vi "UHR-Fleezers Control (host) - Lorentz v5.vi"() -> ()   [LabVIEW 2014] (continued)
            "Current Position" <- w771
            n450 = local write "Stage Control Serial Error"(w774) -> ()
            n451 = Unbundle(w771) -> (w778:dbl, w780:dbl, w776:dbl)
            n452 = Add(x=w780, y="Y change (mm)") -> (x+y=w777:dbl)
            n453 = Bundle(w778, w777, w776) -> (w775:cluster{dbl, dbl, dbl})  [unwired: 1 in]
          }
          frame #1 {
            # "move to new position and start saving"
            n454 = local write "Stage Moving"(TRUE ("Stage Moving")) -> ()
            n455 = local write "Start Saving"(TRUE ("Start Saving")) -> ()
            n456 = call "Set Stage Position.vi"("Position"=w788, "error in"=w787, "VISA resource name in"=w786) -> ("error out"=w784:errorcluster, "VISA resource name out"=w785:refnum<visa-resource-name>)  [unwired: 1 out]
          }
          frame #2 {
            # "go back to start"
            n457 = call "Set Stage Position.vi"("Position"=w790, "error in"=w791, "VISA resource name in"=w792) -> ()  [unwired: 3 out]
          }
          frame #3 {
            # "stop saving"
            n458 = local write "Stop Saving"(TRUE ("Stop Saving")) -> ()
            n459 = local write "Stage Moving"(FALSE ("Stage Moving")) -> ()
          }
        }
      }
      event "Move to Position 1", "Move to Position 2", "Move to Position 3", "Move to Position 4", "Move to Position 5", "Lower Ch. Cap.", "Move to Position 6": Value Change {
        n460 = event-data() -> ()  [unwired: 1 in, 5 out]
        n461 = Or(x="Move to Position 5", y="Lower Ch. Cap.") -> (x .or. y?=w799:bool)
        n462 = Build Array("Move to Position 1", "Move to Position 2", "Move to Position 3", "Move to Position 4", w799, "Move to Position 6") -> (w802:bool[])
        n463 = Boolean Array To Number(Boolean array=w802) -> (number=w801:u32)
        n464 = Logarithm Base 2(1:w801) -> (0:w800:dbl)
        n465 = flat-sequence {
          tunnel: w800 -> [w811]
          tunnel: w797 -> [w809]
          tunnel: w796 -> [w808]
          frame #0 {
            n466 = local read "Saved Stage Positions"() -> (w819:dbl[][])
            n467 = Array Subset(array=w819, index (row)=w811, length (row)=1 ("length"), index (col)=1 ("index"), length (col)=3 ("length")) -> (w816:dbl[][])
            n468 = Reshape Array(w816, 3 ("dimension size")) -> (w814:dbl[])
            n469 = Array To Cluster(array=w814) -> (cluster=w813:cluster{"[0]":dbl, "[1]":dbl, "[2]":dbl})
            n470 = call "Set Stage Position.vi"("Position"=w813, "error in"=w808, "VISA resource name in"=w809) -> ("error out"=w812:errorcluster)  [unwired: 2 out]
            n471 = local write "Stage Moving"(TRUE ("Stage Moving")) -> ()
            n472 = local write "Stage Control Serial Error"(w812) -> ()
          }
          frame #1 {
            n473 = local write "Stage Moving"(FALSE ("Stage Moving")) -> ()
            n474 = call <vilib>:"Beep.vi"() -> ()  [unwired: 3 in, 9 out]
          }
        }
      }
      event "Got Bead 1": Value Change {
        n475 = event-data() -> ()  [unwired: 1 in, 5 out]
        n476 = flat-sequence {
          tunnel: w822 -> [w824]
          tunnel: w822 -> [w828]
          frame #0 {
            n477 = for {
              N: w824 -> [_]
              n478 = property on="Pressure Up" class="Bool (strict)"("Val(Sgnl)"=TRUE) -> ()  [unwired: 2 in, 2 out]
            }
          }
          frame #1 {
          }
          frame #2 {
            n479 = Wait (ms)(milliseconds to wait=u32 1000) -> ()  [unwired: 1 out]
          }
          frame #3 {
          }
          frame #4 {
            n480 = Multiply(x=w828, y=2) -> (x*y=w827:i32)
            n481 = for {
              N: w827 -> [_]
              n482 = property on="Vent pressure" class="Bool (strict)"("Val(Sgnl)"=TRUE) -> ()  [unwired: 2 in, 2 out]
            }
          }
          frame #5 {
            n483 = for {
              N: "Number of Pulses for bead 2" -> [_]
              n484 = property on="Pressure Up" class="Bool (strict)"("Val(Sgnl)"=TRUE) -> ()  [unwired: 2 in, 2 out]
            }
          }
        }
        n485 = local read "Number of pulses For laminar flow"() -> (w822:i32)
      }
      event "Force FB Data\nScript": Value Change {
        n486 = event-data() -> ()  [unwired: 1 in, 5 out]
        n487 = flat-sequence {
          tunnel: w838 -> [w842]
          tunnel: w839 -> [w843]
          tunnel: [w843] -> w834
          tunnel: [w842] -> w833
          tunnel: w834 -> [w846]
          tunnel: w833 -> [w845]
          tunnel: ["Trap Trig Fl."] -> w835
          tunnel: [w871] -> w836
          tunnel: w835 -> [w871]
          tunnel: [w875] -> w837
          tunnel: w836 -> [w875]
          tunnel: w837 -> [w877]
          frame #0 {
            n488 = property on="Trap Delta (MHz)" class="DigNum (strict)"("Val(Sgnl)"="Trap Delta Before Moving") -> ()  [unwired: 2 in, 2 out]
          }
          frame #1 {
            n489 = local read "Saved Stage Positions"() -> (w848:dbl[][])
            n490 = property on="Trap Pos. FB Offset Factor" class="DigNum (strict)"("Val(Sgnl)"=i64 0 ("Value (Signaling)")) -> ()  [unwired: 2 in, 2 out]
            n491 = local write "FB Trap Pos Offset"(0.0 ("FB Trap Pos Offset")) -> ()
            n492 = local write "Stage Moving"(TRUE ("Stage Moving")) -> ()
            n493 = call "move to saved stage position.vi"("error in"=w845, "Stage VISA resource name in"=w846, "Position"="Stage Position To Establish FB", "Saved Stage Positions"=w848) -> ("error out"=w844:errorcluster)  [unwired: 1 out]
            n494 = local write "Stage Control Serial Error"(w844) -> ()
          }
          frame #2 {
            n495 = call <vilib>:"Beep.vi"() -> ()  [unwired: 3 in, 9 out]
            n496 = Multiply(x="Wait (s)", y=u32 1000 ("milliseconds to wait")) -> (x*y=w855:u32)
            n497 = property on="Trap Delta (MHz)" class="DigNum (strict)"("Val(Sgnl)"="Starting \nTrap Delta (MHz)") -> ()  [unwired: 2 in, 2 out]
            n498 = local write "Stage Moving"(FALSE ("Stage Moving")) -> ()
            n499 = Wait (ms)(milliseconds to wait=w855) -> ()  [unwired: 1 out]
            n500 = property on="Tab Control 2" class="TabCtl (strict)"("Val(Sgnl)"=T11."Feedback on Trap Position" ("Value (Signaling)")) -> ()  [unwired: 2 in, 2 out]
            n501 = property on="Tab Control" class="TabCtl (strict)"("Val(Sgnl)"=T40."Trap Control (RF)" ("Value (Signaling)")) -> ()  [unwired: 2 in, 2 out]
          }
          frame #3 {
            n502 = property on="Set Reading to\nSetpoint" class="Bool (strict)"("Val(Sgnl)"=TRUE ("Value (Signaling)")) -> ()  [unwired: 2 in, 2 out]
            n503 = Wait (ms)(milliseconds to wait=u32 500) -> ()  [unwired: 1 out]
          }
          frame #4 {
            n504 = property on="Trap Pos. FB ON" class="Bool (strict)"("Val(Sgnl)"=TRUE ("Value (Signaling)")) -> ()  [unwired: 2 in, 2 out]
            n505 = Wait (ms)(milliseconds to wait=u32 250) -> ()  [unwired: 1 out]
          }
          frame #5 {
            n506 = case shown="False" "Trap Trig Fl." {
              frame False {
                n507 = case shown="True" "Green ON after FB ON?" {
                  selector: "Green ON after FB ON?" -> [_ w870]
                  frame False {
                  }
                  frame True {
                    n508 = property on="Green Laser ON" class="Bool (strict)"("Val(Sgnl)"=w870) -> ()  [unwired: 2 in, 2 out]
                  }
                }
              }
              frame True {
              }
            }
            n509 = case shown="True" "Remove Action Offset" {
              tunnel: TRUE ("Value (Signaling)") -> [w867 w868]
              frame False {
                n510 = property on="Remove Unwinding Offset" class="Bool (strict)"("Val(Sgnl)"=w867) -> ()  [unwired: 2 in, 2 out]
              }
              frame True {
                n511 = property on="Remove Action Offset" class="Bool (strict)"("Val(Sgnl)"=w868) -> ()  [unwired: 2 in, 2 out]
              }
            }
            n512 = Wait (ms)(milliseconds to wait=u32 250) -> ()  [unwired: 1 out]
          }
          frame #6 {
            n513 = property on="Start Saving" class="Bool (strict)"("Val(Sgnl)"=TRUE ("Value (Signaling)")) -> ()  [unwired: 2 in, 2 out]
            n514 = Wait (ms)(milliseconds to wait=u32 5000) -> ()  [unwired: 1 out]
          }
          frame #7 {
            w874 = TRUE ("Value (Signaling)")
            n515 = property on="Rem fb disp offset" class="Bool (strict)"("Val(Sgnl)"=w874) -> ()  [unwired: 2 in, 2 out]
            n516 = property on="Remove Offset" class="Bool (strict)"("Val(Sgnl)"=w874) -> ()  [unwired: 2 in, 2 out]
            n517 = Wait (ms)(milliseconds to wait=u32 100) -> ()  [unwired: 1 out]
          }
          frame #8 {
            n518 = case shown="True" w877 {
              frame False {
              }
              frame True {
                n519 = local write "Trap Trig. Fl."(TRUE ("Value (Signaling)")) -> ()
              }
            }
          }
          frame #9 {
            n520 = case shown="True" "Start dipping after?" {
              frame False {
              }
              frame True {
                n521 = flat-sequence {
                  frame #0 {
                    n522 = Multiply(x="Delay before dipping (s)", y=1000.0) -> (x*y=w881:dbl)
                    n523 = Wait (ms)(milliseconds to wait=w881) -> ()  [unwired: 1 out]
                  }
                  frame #1 {
                    n524 = property on="Dip for Protein" class="Bool (strict)"("Val(Sgnl)"=TRUE ("Value (Signaling)")) -> ()  [unwired: 2 in, 2 out]
                    n525 = local write "Scripts"(T2."Dipping" ("Scripts")) -> ()
                  }
                }
              }
            }
          }
        }
      }
      event "Fixed Traps Data\nScript": Value Change {
        n526 = event-data() -> ()  [unwired: 1 in, 5 out]
        n527 = flat-sequence {
          frame #0 {
            n528 = case shown="True" "Green ON" {
              frame False {
              }
              frame True {
                n529 = property on="Green Laser ON" class="Bool (strict)"("Val(Sgnl)"=TRUE) -> ()  [unwired: 2 in, 2 out]
              }
            }
            n530 = local write "Offset (nm)"(0.0 ("Offset (nm)")) -> ()
            n531 = property on="Sample Channel\nFlow" class="Bool (strict)"("Val(Sgnl)"=FALSE ("Value (Signaling)")) -> ()  [unwired: 2 in, 2 out]
            n532 = property on="Trap Delta (MHz)" class="DigNum (strict)"("Val(Sgnl)"="Fixed Traps Trap Delta (MHz)") -> ()  [unwired: 2 in, 2 out]
          }
          frame #1 {
            n533 = Wait (ms)(milliseconds to wait=u32 1000) -> ()  [unwired: 1 out]
          }
          frame #2 {
            n534 = local write "Start Saving"(TRUE ("Start Saving")) -> ()
          }
          frame #3 {
            n535 = local read "Bead Sep. Int. Time (s)"() -> (w892:dbl)
            n536 = Multiply(x=w892, y=1000.0) -> (x*y=w894:dbl)
            n537 = Wait (ms)(milliseconds to wait=w894) -> ()  [unwired: 1 out]
          }
          frame #4 {
            n538 = property on="Remove Offset" class="Bool (strict)"("Val(Sgnl)"=TRUE ("Value (Signaling)")) -> ()  [unwired: 2 in, 2 out]
          }
          frame #5 {
            n539 = property on="Dip for Protein" class="Bool (strict)"("Val(Sgnl)"="Start dipping after?") -> ()  [unwired: 2 in, 2 out]
          }
        }
      }
      event "Got Bead 2": Value Change {
        # "Got A Dig bead and Got DNA bead events changes by Ronen to Got bead 1 and Got bead 2, and modified to enable operation of the thorlabs motors."
        n540 = event-data() -> ()  [unwired: 1 in, 5 out]
        n541 = flat-sequence {
          tunnel: w897 -> [w900]
          frame #0 {
            n542 = case shown="True" "Lumicks Flow During Calibration" {
              tunnel: w900 -> [_ w901]
              frame False {
              }
              frame True {
                n543 = for {
                  N: w901 -> [_]
                  n544 = property on="Pressure Up" class="Bool (strict)"("Val(Sgnl)"=TRUE) -> ()  [unwired: 2 in, 2 out]
                }
              }
            }
          }
          frame #1 {
          }
          frame #2 {
            n545 = Wait (ms)(milliseconds to wait=u32 1000) -> ()  [unwired: 1 out]
          }
          frame #3 {
          }
          frame #4 {
            n546 = case shown="True" "Calibrate after bead 2?" {
              frame False {
              }
              frame True {
                n547 = property on="Cal/Data Acq. Spot" class="Bool (strict)"("Val(Sgnl)"=TRUE) -> ()  [unwired: 2 in, 2 out]
              }
            }
          }
        }
        n548 = local read "Number of pulses For laminar flow"() -> (w897:i32)
      }
      event "Get New Beads": Value Change {
        # "Flow Control determines how many pressure increases are given when moving."
        n549 = event-data() -> ()  [unwired: 1 in, 6 out]
        n550 = flat-sequence {
          tunnel: w906 -> [w908]
          tunnel: w906 -> [w912]
          frame #0 {
            n551 = for {
              N: w908 -> [_]
              n552 = property on="Pressure Up" class="Bool (strict)"("Val(Sgnl)"=TRUE) -> ()  [unwired: 2 in, 2 out]
            }
          }
          frame #1 {
          }
          frame #2 {
            n553 = Wait (ms)(milliseconds to wait=u32 1000) -> ()  [unwired: 1 out]
          }
          frame #3 {
          }
          frame #4 {
            n554 = Multiply(x=2, y=w912) -> (x*y=w911:i32)
            n555 = for {
              N: w911 -> [_]
              n556 = property on="Vent pressure" class="Bool (strict)"("Val(Sgnl)"=TRUE) -> ()  [unwired: 2 in, 2 out]
            }
          }
          frame #5 {
            n557 = for {
              N: "Number of pulses for Bead 1" -> [_]
              n558 = property on="Pressure Up" class="Bool (strict)"("Val(Sgnl)"=TRUE) -> ()  [unwired: 2 in, 2 out]
            }
          }
        }
        n559 = local read "Number of pulses For laminar flow"() -> (w906:i32)
      }
      event "Take Stepping Data": Value Change {
        n560 = event-data() -> ()  [unwired: 1 in, 5 out]
        n561 = local read "Save ave N"() -> (w925:dbl)
        n562 = flat-sequence {
          tunnel: w925 -> [w927]
          tunnel: [w927] -> w920
          tunnel: [w929] -> w921
          tunnel: w920 -> [w929]
          tunnel: [w931] -> w922
          tunnel: w921 -> [w931]
          tunnel: [w934] -> w923
          tunnel: w922 -> [w934]
          tunnel: [w936] -> w924
          tunnel: w923 -> [w936]
          tunnel: [w938] -> w918
          tunnel: w924 -> [w938]
          tunnel: w918 -> [w941]
          tunnel: [w941] -> w917
          tunnel: w917 -> [w942]
          tunnel: [w942] -> w919
          tunnel: w919 -> [w948]
          frame #0 {
            n563 = property on="Save ave N" class="DigNum (strict)"("Val(Sgnl)"="Save ave factor") -> ()  [unwired: 2 in, 2 out]
          }
          frame #1 {
            n564 = Wait (ms)(milliseconds to wait=u32 100) -> ()  [unwired: 1 out]
          }
          frame #2 {
            n565 = local read "Offset 2 Start (MHz)"() -> (w933:dbl)
            n566 = property on="Saved AOD Raster Scan Parameter Sets" class="Arr (strict)"("Index Values"=u32[] [2]) -> ()  [unwired: 2 in, 2 out]
            n567 = property on="Trap Delta (MHz)" class="DigNum (strict)"("Val(Sgnl)"=w933) -> ()  [unwired: 2 in, 2 out]
          }
          frame #3 {
            n568 = property on="Load parameters" class="Bool (strict)"("Val(Sgnl)"=TRUE ("Value (Signaling)")) -> ()  [unwired: 2 in, 2 out]
          }
          frame #4 {
            n569 = Wait (ms)(milliseconds to wait=u32 100) -> ()  [unwired: 1 out]
          }
          frame #5 {
            n570 = property on="Trap Raster Scan" class="Bool (strict)"("Val(Sgnl)"=TRUE ("Value (Signaling)")) -> ()  [unwired: 2 in, 2 out]
          }
          frame #6 {
            n571 = Wait (ms)(milliseconds to wait=u32 1000) -> ()  [unwired: 1 out]
          }
          frame #7 {
            n572 = while {
              stop <- w945 stop-if-true
              n573 = local read "Raster Scanning..."() -> (w947:bool)
              n574 = local read "Saving..."() -> (w946:bool)
              n575 = Not(x=w946) -> (.not. x?=w943:bool)
              n576 = Not(x=w947) -> (.not. x?=w944:bool)
              n577 = And(x=w944, y=w943) -> (x .and. y?=w945:bool)
            }
          }
          frame #8 {
            n578 = property on="Save ave N" class="DigNum (strict)"("Val(Sgnl)"=w948) -> ()  [unwired: 2 in, 2 out]
          }
        }
      }
      event "Step Size (nm)": Value Change {
        n579 = event-data() -> ()  [unwired: 1 in, 5 out]
        n580 = flat-sequence {
          frame #0 {
            n581 = property on="Saved AOD Raster Scan Parameter Sets" class="Arr (strict)"("Index Values"=u32[] [1]) -> ()  [unwired: 2 in, 2 out]
          }
          frame #1 {
            n582 = Multiply(x="N Steps", y="Step Size (nm)") -> (x*y=w950:dbl)
            n583 = property on="Scan Speed AOD (nm/s) 2" class="DigNum (strict)"("Value"="Step Size (nm)") -> ()  [unwired: 2 in, 2 out]
            n584 = property on="Step Size AOD (nm) 2" class="DigNum (strict)"("Value"="Step Size (nm)") -> ()  [unwired: 2 in, 2 out]
            n585 = property on="Scan Range AOD (nm) 2" class="DigNum (strict)"("Value"=w950) -> ()  [unwired: 2 in, 2 out]
          }
        }
      }
      event "Take Detection Laser\nImage": Value Change {
        n586 = event-data() -> ()  [unwired: 1 in, 5 out]
        n587 = flat-sequence {
          tunnel: [w978] -> w968
          tunnel: [w977] -> w961
          tunnel: [w976] -> w953
          tunnel: [w981] -> w969
          tunnel: w968 -> [w981]
          tunnel: [w980] -> w962
          tunnel: w961 -> [w980]
          tunnel: [w979] -> w954
          tunnel: w953 -> [w979]
          tunnel: [w985] -> w970
          tunnel: w969 -> [w985]
          tunnel: [w984] -> w963
          tunnel: w962 -> [w984]
          tunnel: [w983] -> w955
          tunnel: w954 -> [w983]
          tunnel: [w991] -> w971
          tunnel: w970 -> [w991]
          tunnel: [w990] -> w964
          tunnel: w963 -> [w990]
          tunnel: [w989] -> w956
          tunnel: w955 -> [w989]
          tunnel: [w995] -> w972
          tunnel: w971 -> [w995]
          tunnel: [w994] -> w965
          tunnel: w964 -> [w994]
          tunnel: [w993] -> w957
          tunnel: w956 -> [w993]
          tunnel: [w999] -> w973
          tunnel: w972 -> [w999]
          tunnel: [w998] -> w966
          tunnel: w965 -> [w998]
          tunnel: [w997] -> w958
          tunnel: w957 -> [w997]
          tunnel: [w1003] -> w974
          tunnel: w973 -> [w1003]
          tunnel: [w1002] -> w967
          tunnel: w966 -> [w1002]
          tunnel: [w1001] -> w959
          tunnel: w958 -> [w1001]
          tunnel: w974 -> [w1009]
          tunnel: w967 -> [w1008]
          tunnel: [w1006] -> w960
          tunnel: w959 -> [w1006]
          tunnel: w960 -> [w1010]
          frame #0 {
            n588 = local read "Laser interlacing mode"() -> (w977:enum32{"Laser ON", "Laser OFF", "Interlace"})
            n589 = local read "Green FB On/Off"() -> (w976:bool)
            n590 = local read "Green Laser ON"() -> (w978:bool)
          }
          frame #1 {
            n591 = property on="Green FB On/Off" class="Bool (strict)"("Val(Sgnl)"=FALSE ("Value (Signaling)")) -> ()  [unwired: 2 in, 2 out]
          }
          frame #2 {
            n592 = property on="Green Laser ON" class="Bool (strict)"("Val(Sgnl)"=TRUE ("Value (Signaling)")) -> ()  [unwired: 2 in, 2 out]
            n593 = property on="Flip Green Filter" class="Bool (strict)"("Val(Sgnl)"=TRUE ("Value (Signaling)")) -> ()  [unwired: 2 in, 2 out]
            n594 = property on="Laser interlacing mode" class="RadioBtnsControl (strict)"("Val(Sgnl)"=enum32{"Laser ON", "Laser OFF", "Interlace"}."Laser ON" ("Value (Signaling)")) -> ()  [unwired: 2 in, 2 out]
          }
          frame #3 {
            n595 = Wait (ms)(milliseconds to wait=u32 500) -> ()  [unwired: 1 out]
          }
          frame #4 {
            n596 = property on="Confocal Image" class="Bool (strict)"("Val(Sgnl)"=TRUE ("Value (Signaling)")) -> ()  [unwired: 2 in, 2 out]
          }
          frame #5 {
            n597 = Wait (ms)(milliseconds to wait=u32 2000) -> ()  [unwired: 1 out]
          }
          frame #6 {
            n598 = while {
              stop <- w1004 stop-if-true
              n599 = local read "Saving..."() -> (w1005:bool)
              n600 = Not(x=w1005) -> (.not. x?=w1004:bool)
            }
          }
          frame #7 {
            n601 = property on="Flip Green Filter" class="Bool (strict)"("Val(Sgnl)"=TRUE ("Value (Signaling)")) -> ()  [unwired: 2 in, 2 out]
            n602 = property on="Green Laser ON" class="Bool (strict)"("Val(Sgnl)"=w1009) -> ()  [unwired: 2 in, 2 out]
            n603 = property on="Laser interlacing mode" class="RadioBtnsControl (strict)"("Val(Sgnl)"=w1008) -> ()  [unwired: 2 in, 2 out]
          }
          frame #8 {
            n604 = property on="Green FB On/Off" class="Bool (strict)"("Val(Sgnl)"=w1010) -> ()  [unwired: 2 in, 2 out]
          }
        }
      }
      event "Move in a Circle": Value Change {
        w1012 = dbl[] []
        # "converting distance (d) to angle (a)\na=arcsin(d/2r)"
        # "radius"
        # "radius"
        # "T1 Y"
        # "T1 X"
        n605 = event-data() -> ()  [unwired: 1 in, 5 out]
        n606 = local read "BD 1 Frequency 1 (MHz)"() -> (w1020:dbl)
        n607 = local read "BD 2 Frequency 1 (MHz)"() -> (w1019:dbl)
        n608 = local read "BD 1 Frequency 2 (MHz)"() -> (w1018:dbl)
        n609 = local read "BD 2 Frequency 2 (MHz)"() -> (w1017:dbl)
        n610 = Subtract(x=w1019, y="Center Y Frequency (MHz)") -> (x-y=w1024:dbl)
        n611 = Absolute Value(x=w1024) -> (abs(x)=w1015:dbl)
        n612 = flat-sequence {
          tunnel: w1015 -> [w1027]
          tunnel: [w1027] -> w1014
          frame #0 {
            n613 = local write "Radius (MHz)"(w1027) -> ()
          }
        }
        n614 = node-c288("Time step (ms)") -> (w1026:T36)  [unwired: 3 in]
        n615 = timed-loop {
          timing: w1026 -> [_]
          timing-out: [_] -> w1025
          tunnel: w1020 -> [w1118]
          tunnel: w1019 -> [_]
          tunnel: w1018 -> [w1122]
          tunnel: w1017 -> [_]
          tunnel: "Center Y Frequency (MHz)" -> [w1111]
          shift-right: [w1072] -> _
          shift-left: w1012 -> [w1079]
          shift-right: [w1070] -> _
          shift-left: w1012 -> [w1078]
          shift-right: [w1063] -> _
          shift-left: w1012 -> [w1076]
          shift-right: [w1061] -> _
          shift-left: w1012 -> [w1075]
          tunnel: "Move in a Circle" -> [_]
          tunnel: ["Back to start on finish?"] -> w1016
          tunnel: w1014 -> [_]
          tunnel: w1013 -> [w1093]
          tunnel: w1012 -> [w1074]
          shift-right: [w1045] -> _
          shift-left: 0.0 -> [w1043]
          i -> [w1052]
          stop <- w1116 stop-if-true
          w1060 = 0 ("index")
          w1081 = 1 ("dimension size")
          # "Keep phase within\n2pi so errors don't \nbuild"
          # "Accumulated\nphase"
          # "Current phase"
          # "Trap 2"
          # "Trap 1"
          # "ignore if N = 0"
          # "r"
          # "r"
          # "r"
          # "r"
          # "\"omega*t\""
          # "Trap 2"
          # "Trap separation (radians)"
          # "Trap 1"
          # "Offset (starts\n at bottom of\n the circle)"
          # "omega"
          n616 = node-c288() -> (w1129:i64)  [unwired: 1 in]
          n617 = Divide(x=w1129, y=1000) -> (x/y=w1048:dbl)
          n618 = Divide(x="2D Motion Trap Separation (MHz)", y="Radius (MHz)") -> (x/y=w1103:dbl)
          n619 = Negate(x=w1048) -> (-x=w1047:dbl)
          n620 = Divide(x="Trap 2 phase shift (deg)", y=360.0) -> (x/y=w1094:dbl)
          n621 = Inverse Sine(1:w1103) -> (0:w1039:dbl)
          n622 = Multiply(x=6.283185307179586, y=w1094) -> (x*y=w1040:dbl)
          n623 = Multiply(x=6.283185307179586, y="2D Motion Frequency (Hz)") -> (x*y=w1051:dbl)
          n624 = Select(t=w1048, s="Counterclockwise/Clockwise", f=w1047) -> (s? t:f=w1050:dbl)
          n625 = Multiply(x=w1051, y=w1050) -> (x*y=w1041:dbl)
          n626 = Select(t=w1039, s="Trap shift\nmethod", f=w1040) -> (s? t:f=w1038:dbl)
          n627 = Add(x=w1041, y=w1043) -> (x+y=w1044:dbl)
          n628 = Add(x=w1044, y=w1038) -> (x+y=w1100:dbl)
          n629 = Add(x=w1044, y=1.5707963267948966) -> (x+y=w1049:dbl)
          n630 = Add(x=w1100, y=1.5707963267948966) -> (x+y=w1113:dbl)
          n631 = Cosine(x=w1049) -> (cos(x)=w1127:dbl)
          n632 = Sine(x=w1049) -> (sin(x)=w1126:dbl)
          n633 = Multiply(x=w1127, y="Radius (MHz)") -> (x*y=w1120:dbl)
          n634 = Cosine(x=w1113) -> (cos(x)=w1125:dbl)
          n635 = Sine(x=w1113) -> (sin(x)=w1124:dbl)
          n636 = Multiply(x=w1126, y="Radius (MHz)") -> (x*y=w1119:dbl)
          n637 = Multiply(x=w1125, y="Radius (MHz)") -> (x*y=w1123:dbl)
          n638 = Multiply(x=w1124, y="Radius (MHz)") -> (x*y=w1121:dbl)
          n639 = Add(x=w1120, y=w1118) -> (x+y=w1069:dbl)
          n640 = Add(x=w1119, y=w1111) -> (x+y=w1067:dbl)
          n641 = Greater Or Equal?(x=w1052, y="N steps then stop") -> (x >= y?=w1110:bool)
          n642 = Add(x=w1123, y=w1122) -> (x+y=w1058:dbl)
          n643 = Add(x=w1121, y=w1111) -> (x+y=w1056:dbl)
          n644 = Not Equal To 0?(x="N steps then stop") -> (x != 0?=w1106:bool)
          n645 = And(x=w1110, y=w1106) -> (x .and. y?=w1107:bool)
          n646 = local read "Trap 1 sum mean"() -> (w1090:dbl)
          n647 = local read "Stop All"() -> (w1115:bool)
          n648 = local write "BD 1 Frequency 1 (MHz)"(w1069) -> ()
          n649 = local write "BD 2 Frequency 1 (MHz)"(w1067) -> ()
          n650 = local write "BD 1 Frequency 2 (MHz)"(w1058) -> ()
          n651 = local write "BD 2 Frequency 2 (MHz)"(w1056) -> ()
          n652 = Select(t=w1052, s="test", f=w1090) -> (s? t:f=→"Waveform Chart":dbl)
          n653 = Compound Arithmetic op=OR(w1115, "Stop Moving", w1107) -> (w1116:bool)
          n654 = local read "BD 1 Frequency 3 (MHz)"() -> (w1099:dbl)
          n655 = local read "BD 2 Frequency 3 (MHz)"() -> (w1098:dbl)
          n656 = Select(t=w1074, s="Reset graph", f=w1075) -> (s? t:f=w1055:dbl[])
          n657 = Select(t=w1074, s="Reset graph", f=w1076) -> (s? t:f=w1057:dbl[])
          n658 = Select(t=w1074, s="Reset graph", f=w1078) -> (s? t:f=w1066:dbl[])
          n659 = Select(t=w1074, s="Reset graph", f=w1079) -> (s? t:f=w1068:dbl[])
          n660 = Initialize Array(w1056, w1081) -> (w1082:dbl[])
          n661 = Initialize Array(w1067, w1081) -> (w1085:dbl[])
          n662 = Initialize Array(w1058, w1081) -> (w1083:dbl[])
          n663 = Initialize Array(w1069, w1081) -> (w1086:dbl[])
          n664 = local read "Y RF Frequency Limits (MHz)"() -> (w1096:T23)
          n665 = local read "X RF Frequency Limits (MHz)"() -> (w1097:T23)
          n666 = call "set RF board frequency - interlace.vi"("Board 2 Frequency Limits"=w1096, "Board 1 Frequency Limits"=w1097, "FPGA VI Reference In"=w1093, "Board 2 Frequency 3 (MHz)"=w1098, "Board 1 Frequency 3 (MHz)"=w1099, "Board 2 Frequency 2 (MHz)"=w1056, "Board 2 Frequency 1 (MHz)"=w1067, "Board 1 Frequency 2 (MHz)"=w1058, "Board 1 Frequency 1  (MHz)"=w1069) -> ()  [unwired: 1 in, 2 out]
          n667 = Bundle(w1083, w1082) -> (w1054:cluster{dbl[], dbl[]})  [unwired: 1 in]
          n668 = Bundle(w1086, w1085) -> (w1084:cluster{dbl[], dbl[]})  [unwired: 1 in]
          n669 = Build Array (concatenate)(w1069, w1068) -> (w1073:dbl[])
          n670 = Build Array (concatenate)(w1067, w1066) -> (w1071:dbl[])
          n671 = Build Array (concatenate)(w1058, w1057) -> (w1064:dbl[])
          n672 = Build Array (concatenate)(w1056, w1055) -> (w1062:dbl[])
          n673 = Bundle(w1073, w1071) -> (w1053:cluster{dbl[], dbl[]})  [unwired: 1 in]
          n674 = Bundle(w1064, w1062) -> (w1080:cluster{dbl[], dbl[]})  [unwired: 1 in]
          n675 = Build Array(w1084, w1054, w1053, w1080) -> (→"Trap trajectories":cluster{dbl[], dbl[]}[])
          n676 = case "To pause the process" shown="True" "Pause rotation" {
            frame False {
            }
            frame True {
              n677 = while {
                stop <- w1132 stop-if-true
                n678 = local read "Pause rotation"() -> (w1133:bool)
                n679 = Wait (ms)(milliseconds to wait=u32 10) -> ()  [unwired: 1 out]
                n680 = Not(x=w1133) -> (.not. x?=w1132:bool)
              }
            }
          }
          n681 = Decrement(x="N steps to plot") -> (x-1=w1059:i32)
          n682 = Array Subset(array=w1071, index=w1060, length=w1059) -> (w1070:dbl[])
          n683 = Array Subset(array=w1073, index=w1060, length=w1059) -> (w1072:dbl[])
          n684 = Array Subset(array=w1064, index=w1060, length=w1059) -> (w1063:dbl[])
          n685 = Array Subset(array=w1062, index=w1060, length=w1059) -> (w1061:dbl[])
          n686 = Quotient & Remainder(x=w1044, y=6.283185307179586) -> (x-y*floor(x/y)=w1045:dbl)  [unwired: 1 out]
          n687 = node-c288() -> ()  [unwired: 1 in, 1 out]
        }
        n688 = node-c288(w1025) -> ()  [unwired: 1 out]
        n689 = case shown="True" w1016 {
          tunnel: w1020 -> [_ w1031]
          tunnel: w1019 -> [_ w1030]
          tunnel: w1018 -> [_ w1029]
          tunnel: w1017 -> [_ w1028]
          frame False {
          }
          frame True {
            n690 = flat-sequence {
              tunnel: w1031 -> [w1035]
              tunnel: w1030 -> [w1034]
              tunnel: w1029 -> [w1033]
              tunnel: w1028 -> [w1032]
              frame #0 {
                n691 = local write "BD 1 Frequency 1 (MHz)"(w1035) -> ()
                n692 = local write "BD 2 Frequency 1 (MHz)"(w1034) -> ()
                n693 = local write "BD 1 Frequency 2 (MHz)"(w1033) -> ()
                n694 = local write "BD 2 Frequency 2 (MHz)"(w1032) -> ()
              }
              frame #1 {
                n695 = property on="Update all trap values" class="Bool (strict)"("Val(Sgnl)"=TRUE ("Value (Signaling)")) -> ()  [unwired: 2 in, 2 out]
              }
            }
          }
        }
      }
      event "Stop All": Value Change {
        # "Stopping blue laser before shutting off program"
        n696 = event-data() -> ()  [unwired: 1 in, 5 out]
        n697 = local read "Delay (ms)"() -> (w1143:i32)
        n698 = call "serial write macro.vi"("String"="l0", "Delay (ms)"=w1143, "VISA resource name"=w1146) -> ("read buffer"=w1141:string, "error out"=w1142:errorcluster, "VISA resource name out"=w1145:refnum<visa-resource-name>)
        n699 = local write "read blue buffer"(w1141) -> ()
        n700 = local write "Blue Error Out"(w1142) -> ()
        n701 = VISA Close(VISA resource name=w1145) -> ()  [unwired: 1 in, 1 out]
        n702 = local read "Stop All"() -> (w1147:bool)
      }
      event "Sensitivity", "Offset Current Sign", "Offset Current Value", "Offset Current", "Bias Voltage", "Bias Voltage (mV)", "Filter Type", "Lowpass 3dB Point", "Highpass 3dB Point", "Filter Reset", "Invert Signal", "Gain Mode", "Send Command": Value Change {
        w1154 = 250 ("Delay (ms)")
        n703 = event-data() -> ()  [unwired: 1 in, 5 out]
        n704 = event shown="[0] \"Sensitivity\": Value Change" {
          selector: _ -> [_ _ _ _ _ _ _ _ _ _ _ _ _]
          dyn-events: _ -> [_ _ _ _ _ _ _ _ _ _ _ _ _]
          timeout: _ -> [_ _ _ _ _ _ _ _ _ _ _ _ _]
          tunnel: [w1166 w1174 w1182 w1191 w1201 w1209 w1212 w1216 w1219 w1222 w1225 w1232 "Command"] -> w1153
          tunnel: [w1161 w1168 w1178 w1185 w1195 w1205 _ _ _ _ _ w1228 _] -> w1148
          event "Sensitivity": Value Change {
            n705 = event-data() -> ()  [unwired: 1 in, 5 out]
            n706 = property on="Sensitivity" class="CmbBox"() -> ("Value"=→"Gain":string)  [unwired: 2 in, 2 out]
            n707 = Concatenate Strings("SENS ", "Sensitivity") -> (w1166:string)
            n708 = local read "Gain"() -> (w1163:string)
            n709 = Concatenate Strings("gain set at ", w1163) -> (w1161:string)
          }
          event "Offset Current Sign": Value Change {
            n710 = event-data() -> ()  [unwired: 1 in, 4 out]
            n711 = Boolean To (0,1)(Boolean="Offset Current Sign") -> (0, 1=w1177:i16)
            n712 = Select(t="positive", s="Offset Current Sign", f="negative") -> (s? t:f=w1169:string)
            n713 = Number To Decimal String(number=w1177) -> (decimal integer string=w1176:string)  [unwired: 1 in]
            n714 = Concatenate Strings("IOSN " ("string"), w1176) -> (w1174:string)
            n715 = Concatenate Strings("offset current sign ", w1169) -> (w1168:string)
          }
          event "Offset Current Value": Value Change {
            n716 = event-data() -> ()  [unwired: 1 in, 5 out]
            n717 = property on="Offset Current Value" class="CmbBox"() -> ("Value"=→"Read offset current":string)  [unwired: 2 in, 2 out]
            n718 = local read "Read offset current"() -> (w1179:string)
            n719 = Concatenate Strings("IOLV ", "Offset Current Value") -> (w1182:string)
            n720 = Concatenate Strings("offset current value ", w1179) -> (w1178:string)
          }
          event "Offset Current": Value Change {
            n721 = event-data() -> ()  [unwired: 1 in, 5 out]
            n722 = Boolean To (0,1)(Boolean="Offset Current") -> (0, 1=w1194:i16)
            n723 = Select(t="on", s="Offset Current", f="off") -> (s? t:f=w1186:string)
            n724 = Number To Decimal String(number=w1194) -> (decimal integer string=w1193:string)  [unwired: 1 in]
            n725 = Concatenate Strings("IOON " ("string"), w1193) -> (w1191:string)
            n726 = Concatenate Strings("offset current ", w1186) -> (w1185:string)
          }
          event "Bias Voltage": Value Change {
            n727 = event-data() -> ()  [unwired: 1 in, 5 out]
            n728 = Boolean To (0,1)(Boolean="Bias Voltage") -> (0, 1=w1202:i16)
            n729 = Number To Decimal String(number=w1202) -> (decimal integer string=w1203:string)  [unwired: 1 in]
            n730 = Select(t="on", s="Bias Voltage", f="off") -> (s? t:f=w1196:string)
            n731 = Concatenate Strings("BSON " ("string"), w1203) -> (w1201:string)
            n732 = Concatenate Strings("bias voltage", w1196) -> (w1195:string)
          }
          event "Bias Voltage (mV)": Value Change {
            n733 = event-data() -> ()  [unwired: 1 in, 5 out]
            n734 = Number To Decimal String(number="Bias Voltage (mV)") -> (decimal integer string=w1211:string)  [unwired: 1 in]
            n735 = Number To Fractional String(number="Bias Voltage (mV)") -> (F-format string=w1206:string)  [unwired: 3 in]
            n736 = Concatenate Strings("BSLV " ("string"), w1211) -> (w1209:string)
            n737 = Concatenate Strings("bias voltage value ", w1206) -> (w1205:string)
          }
          event "Filter Type": Value Change {
            n738 = event-data() -> ()  [unwired: 1 in, 5 out]
            n739 = Concatenate Strings("FLTT " ("string"), "Filter Type") -> (w1212:string)
          }
          event "Lowpass 3dB Point": Value Change {
            n740 = event-data() -> ()  [unwired: 1 in, 5 out]
            n741 = Concatenate Strings("LFRQ " ("string"), "Lowpass 3dB Point") -> (w1216:string)
          }
          event "Highpass 3dB Point": Value Change {
            n742 = event-data() -> ()  [unwired: 1 in, 5 out]
            n743 = Concatenate Strings("HFRQ " ("string"), "Highpass 3dB Point") -> (w1219:string)
          }
          event "Filter Reset": Value Change {
            n744 = event-data() -> ()  [unwired: 1 in, 5 out]
            n745 = Select(t="ROLD", s="Filter Reset", f="") -> (s? t:f=w1222:string)
          }
          event "Gain Mode": Value Change {
            n746 = event-data() -> ()  [unwired: 1 in, 5 out]
            n747 = Concatenate Strings("GNMD " ("string"), "Gain Mode") -> (w1225:string)
          }
          event "Invert Signal": Value Change {
            n748 = event-data() -> ()  [unwired: 1 in, 5 out]
            n749 = Boolean To (0,1)(Boolean="Invert Signal") -> (0, 1=w1235:i16)
            n750 = Number To Decimal String(number=w1235) -> (decimal integer string=w1234:string)  [unwired: 1 in]
            n751 = Concatenate Strings("INVT " ("string"), w1234) -> (w1232:string)
            n752 = Select(t="signal inverted", s="Invert Signal", f="signal not inverted") -> (s? t:f=w1228:string)
          }
          event "Send Command": Value Change {
            n753 = event-data() -> ()  [unwired: 1 in, 5 out]
          }
        }
        "Command Sent" <- w1153
        n754 = local read "Save Event Log?"() -> (w1149:bool)
        n755 = local read "Saving..."() -> (w1150:bool)
        n756 = And(x=w1149, y=w1150) -> (x .and. y?=w1151:bool)
        n757 = case shown="True" w1151 {
          tunnel: w1148 -> [_ w1158]
          frame False {
          }
          frame True {
            n758 = local read "Time (s)"() -> (w1159:dbl)
            n759 = local read "log file ref"() -> (w1160:refnum<file>)
            n760 = call "write to event log.vi"("log file ref"=w1160, "time"=w1159, "input string"=w1158) -> ()  [unwired: 8 in]
          }
        }
        n761 = call "preamp serial write macro.vi"("String"=w1153, "Delay (ms)"=w1154, "VISA resource name"=w1157) -> ("read buffer"=→"Reply":string, "error out"=w1156:errorcluster)  [unwired: 1 out]
        n762 = call "preamp serial write macro.vi"("String"=w1153, "Delay (ms)"=w1154, "VISA resource name"=w1152) -> ()  [unwired: 3 out]
        n763 = local write "Preamp Error Out"(w1156) -> ()
      }
    }
    n764 = node-c288() -> ()  [unwired: 1 in, 1 out]
  }
  n765 = flat-sequence "Safety limits on RF frequencies and amplitudes (for AOM protection)" {
    tunnel: [w1239] -> w17
    tunnel: [w1237] -> w19
    tunnel: [w1240] -> w20
    tunnel: [w1241] -> w18
    tunnel: w1 -> [w1239]
    tunnel: T23 {"Minimum"=0.0, "Maximum"=50.0, "Increment"=1.0} ("Data Entry Limits") -> [w1237]
    tunnel: w6 -> [w1238]
    tunnel: [w1238] -> w21
    frame #0 {
      w1241 = T23 {"Minimum"=0.0, "Maximum"=40.0, "Increment"=0.1} ("Min Max Inc")
      w1240 = T23 {"Minimum"=0.0, "Maximum"=45.0, "Increment"=1.0} ("Data Entry Limits")
      n766 = property on="BD 2 Frequency 1 (MHz)" class="DigNum (strict)"("Data Range"=w1241) -> ()  [unwired: 2 in, 2 out]
      n767 = property on="BD 2 Frequency 3 (MHz)" class="DigNum (strict)"("Data Range"=w1241) -> ()  [unwired: 2 in, 2 out]
      n768 = property on="BD 2 Frequency 2 (MHz)" class="DigNum (strict)"("Data Range"=w1241) -> ()  [unwired: 2 in, 2 out]
      n769 = property on="BD 1 Frequency 1 (MHz)" class="DigNum (strict)"("Data Range"=w1239) -> ()  [unwired: 2 in, 2 out]
      n770 = property on="BD 1 Frequency 2 (MHz)" class="DigNum (strict)"("Data Range"=w1239) -> ()  [unwired: 2 in, 2 out]
      n771 = property on="BD 1 Frequency 3 (MHz)" class="DigNum (strict)"("Data Range"=w1239) -> ()  [unwired: 2 in, 2 out]
      n772 = property on="BD 2 Amplitude 1 (%)" class="DigNum (strict)"("Data Range"=w1240) -> ()  [unwired: 2 in, 2 out]
      n773 = property on="BD 2 Amplitude 2 (%)" class="DigNum (strict)"("Data Range"=w1240) -> ()  [unwired: 2 in, 2 out]
      n774 = property on="BD 2 Amplitude 3 (%)" class="DigNum (strict)"("Data Range"=w1240) -> ()  [unwired: 2 in, 2 out]
      n775 = property on="BD 1 Amplitude 3 (%)" class="DigNum (strict)"("Data Range"=w1237) -> ()  [unwired: 2 in, 2 out]
      n776 = property on="BD 1 Amplitude 2 (%)" class="DigNum (strict)"("Data Range"=w1237) -> ()  [unwired: 2 in, 2 out]
      n777 = property on="BD 1 Amplitude 1 (%)" class="DigNum (strict)"("Data Range"=w1237) -> ()  [unwired: 2 in, 2 out]
      "X RF Frequency Limits (MHz)" <- w1239
      "X RF Amplitude Limits (%)" <- w1237
      "Y RF Amplitude Limits (%)" <- w1240
      "Y RF Frequency Limits (MHz)" <- w1241
    }
  }
  n778 = stacked-sequence "Host initialization sequence - order matters!" {
    tunnel: w21 -> [_ w1261 w1353 _ w1410 w1419 w1486 w1510 _ w1553]
    tunnel: [_ _ _ _ _ _ _ _ _ w1553] -> w10
    tunnel: [_ _ _ _ _ _ _ _ _ w1552] -> w23
    tunnel: w20 -> [_ _ _ _ _ _ w1484 _ _ _]
    tunnel: w19 -> [_ _ _ _ _ _ w1483 _ _ _]
    tunnel: w18 -> [_ _ _ _ _ _ w1482 _ _ _]
    tunnel: w17 -> [_ _ _ _ _ _ w1463 _ _ _]
    tunnel: [_ _ _ _ _ _ _ _ w1550 _] -> _
    frame #0 {
    }
    frame #1 {
      w1293 = 10.0 ("y")
      w1294 = 32767.0 ("y")
      w1278 = 6.0  # clock mult.
      w1277 = 49152000.0  # TCXO frequ.
      # "Initialize some FPGA settings"
      n779 = local read "Not-Interlacing Set"() -> (w1333:enum32{"Set 1", "Set 2", "Set 3"})
      n780 = local write "Trap Pos FIFO Timeout"(u16 0 ("Trap Pos FIFO Timeout")) -> ()
      n781 = local read "Interlace"() -> (w1331:bool)
      n782 = local read "Desired Scan Incr (V)"() -> (w1305:dbl)
      n783 = local read "BD 1 Delay (ticks)"() -> (w1340:u8)
      n784 = local read "Number Interlace Sets"() -> (w1332:u8)
      n785 = local read "BD 2 Delay (Ticks)"() -> (w1341:u8)
      n786 = property on="AI Count (ticks)" class="DigNum (strict)"("Val(Sgnl)"="AI Count (ticks)") -> ()  [unwired: 2 in, 2 out]
      n787 = local read "AO1"() -> (w1299:dbl)
      n788 = local read "AO2"() -> (w1300:dbl)
      n789 = local read "Next trap write delay (ticks)"() -> (w1342:u8)
      n790 = local read "Number of scans (MCL)"() -> (w1309:u64)
      n791 = local read "Cycles/step (MCL)"() -> (w1308:u64)
      n792 = local read "Scan steps (MCL)"() -> (w1307:u64)
      n793 = local read "Continuous MCL Scanning"() -> (w1310:bool)
      n794 = Multiply(x=w1299, y=w1294) -> (x*y=w1297:dbl)
      n795 = Multiply(x=w1300, y=w1294) -> (x*y=w1295:dbl)
      n796 = Build Array("DIO count 1 (ticks)", "DIO count 2 (ticks)", "DIO count 3 (ticks)") -> (w1326:u16[])
      n797 = local read "Fast Scan Dir"() -> (w1311:bool)
      n798 = local read "2D or 1D Scan"() -> (w1323:bool)
      n799 = local read "N Acq Sets (Traps + Fl.)"() -> (w1319:i16)
      n800 = local read "Scan Increment (MHz)"() -> (w1282:dbl)
      n801 = Divide(x=w1297, y=w1293) -> (x/y=w1298:dbl)
      n802 = Divide(x=w1295, y=w1293) -> (x/y=w1296:dbl)
      n803 = To Unsigned Byte Integer(number=w1333) -> (unsigned 8bit integer=w1328:u8)
      n804 = Split 1D Array(array=w1326, index=w1332) -> (first subarray=w1324:u16[])  [unwired: 1 out]
      n805 = Multiply(x=w1305, y=32767.0) -> (x*y=w1303:dbl)
      n806 = To Word Integer(number=w1298) -> (16bit integer=w1244:i16)
      n807 = To Word Integer(number=w1296) -> (16bit integer=w1243:i16)
      n808 = Index Array(array=w1326, index=w1328) -> (element=w1327:u16)
      n809 = Add Array Elements(numeric array=w1324) -> (sum=w1325:u16)
      n810 = Multiply(x=w1277, y=w1278) -> (x*y=w1279:dbl)
      n811 = Divide(x=w1303, y=10.0) -> (x/y=w1304:dbl)
      n812 = Select(t=w1325, s=w1331, f=w1327) -> (s? t:f=w1334:u16)
      n813 = Not(x=w1311) -> (.not. x?=w1312:bool)
      n814 = To Word Integer(number=w1304) -> (16bit integer=w1306:i16)
      n815 = property on="2D or 1D Scan" class="Bool (strict)"("Val(Sgnl)"=w1323) -> ()  [unwired: 2 in, 2 out]
      n816 = Divide(x=40000000.0, y="AI Count (ticks)") -> (x/y=w1315:dbl)
      n817 = local write "Update Count (MCL)"(w1334) -> ()
      n818 = local write "Total Counts (ticks)"(w1334) -> ()
      n819 = Divide(x=w1315, y="FPGA Ave.") -> (x/y=w1314:dbl)
      n820 = local write "AI rate (Hz)"(w1315) -> ()
      n821 = Multiply(x=w1282, y=1000.0) -> (x*y=w1275:dbl)
      n822 = local write "Ave. Rate (Hz)"(w1314) -> ()
      n823 = Reciprocal(x=w1314) -> (1/x=w1313:dbl)
      n824 = Scale By Power Of 2(n=48, x=w1275) -> (x*2^n=w1274:dbl)
      n825 = local write "Ave. Period (s)"(w1313) -> ()
      n826 = Divide(x=w1274, y=w1279) -> (x/y=w1280:dbl)
      n827 = To Quad Integer(1:w1280) -> (0:w1283:i64)
      n828 = local read "Setpoints (V)"() -> (w1268:cluster{"Set 1":dbl, "Set 2":dbl})
      n829 = local read "# Samples/channel"() -> (w1290:u32)
      n830 = local read "Feedback On/Off"() -> (w1265:cluster{"Set 1":bool, "Set 2":bool})
      n831 = local read "T3 Y (V)"() -> (w1248:dbl)
      n832 = local read "T3 X (V)"() -> (w1247:dbl)
      n833 = local read "Trap intensity output range"() -> (w1258:cluster{"Normal High":i16, "Normal Low":i16})
      n834 = local read "All FB On/Off"() -> (w1264:bool)
      n835 = local read "Number of F/B Scans (AOD)"() -> (w1289:u16)
      n836 = local read "Trap Intensity PID Gains"() -> (w1257:T14)
      n837 = local read "Cycles/step (AOD)"() -> (w1285:u64)
      n838 = local read "Scan steps (AOD)"() -> (w1284:u64)
      n839 = Multiply(x=w1284, y=w1285) -> (x*y=w1286:u64)
      n840 = Multiply(x=w1286, y=u64 2) -> (x*y=w1288:u64)
      n841 = Multiply(x=w1288, y=w1289) -> (x*y=w1291:u64)
      n842 = Multiply(x=3276.7, y=w1268) -> (x*y=w1269:cluster{"Set 1":dbl, "Set 2":dbl})
      n843 = local read "Scan BD"() -> (w1273:bool)
      n844 = Multiply(x=w1248, y=32767.0) -> (x*y=w1254:dbl)
      n845 = And(x=w1265, y=w1264) -> (x .and. y?=w1266:cluster{"Set 1":bool, "Set 2":bool})
      n846 = To Word Integer(number=w1269) -> (16bit integer=w1270:cluster{"Set 1":i16, "Set 2":i16})
      n847 = Multiply(x=w1247, y=32767.0) -> (x*y=w1251:dbl)
      n848 = local read "Sets to FIFO (Traps)"() -> (w1336:T22)
      n849 = Divide(x=w1291, y=w1290) -> (x/y=w1292:dbl)
      n850 = Unbundle By Name(w1266) -> ("Set 1"=w1262:bool, "Set 2"=w1263:bool)
      n851 = Unbundle By Name(w1270) -> ("Set 1"=w1271:i16, "Set 2"=w1272:i16)
      n852 = Divide(x=w1254, y=10.0) -> (x/y=w1255:dbl)
      n853 = Divide(x=w1251, y=10.0) -> (x/y=w1250:dbl)
      n854 = To Unsigned Word Integer(number=w1255) -> (unsigned 16bit integer=w1246:u16)
      n855 = To Unsigned Word Integer(number=w1250) -> (unsigned 16bit integer=w1245:u16)
      n856 = local read "FPGA error out"() -> (w1260:errorcluster)
      n857 = local write "Data points/scan (f/b)"(w1288) -> ()
      n858 = local write "Data points/scans"(w1291) -> ()
      n859 = local write "N sets should be saved"(w1292) -> ()
      n860 = Unbundle By Name(w1336) -> ("Set 1"=w1337:bool, "Set 2"=w1338:bool, "Set 3"=w1339:bool)
      n861 = xnode "Read/Write Control"("FPGA VI Reference In"=w1261, "error in"=w1260, "ai count"="AI Count (ticks)", "Interlace ON/OFF"=w1331, "Number Interlace Cycles"=w1332, "Set 1"=w1337, "Set 2"=w1338, "Set 3"=w1339, "FB On/Off Set 1"=w1262, "FB On/Off Set 2"=w1263, "Interlace Off Parameters"=w1333, "FB Setpoint Set 1"=w1271, "FB Setpoint Set 2"=w1272, "Piezo Trap Y (AO4)"=w1246, "Piezo Trap X (AO5)"=w1245, "FB Gains"=w1257, "FB output range"=w1258, "Cycles per step"=w1285, "Scan BD"=w1273, "Number of scans"=w1289, "Scan steps"=w1284, "Scan freq.  increment"=w1283, "AO1"=w1244, "AO2"=w1243, "Scan freq.  increment (MCL)"=w1306, "Scan steps (MCL)"=w1307, "Cycles per step (MCL)"=w1308, "Number of scans (MCL)"=w1309, "MCL count"=w1334, "Cont. Scan (MCL)"=w1310, "MCL Scan Axis"=w1312, "1D or 2D Scan?"=w1323, "N of AI1 Int Acq Sets"=w1319, "Amp switch delay"="Amp switch delay", "Swap F1 and F2"="Swap F1 and F2", "APD to FIFO"=FALSE, "DIO count 1 (ticks)"="DIO count 1 (ticks)", "DIO count 2 (ticks)"="DIO count 2 (ticks)", "DIO count 3 (ticks)"="DIO count 3 (ticks)", "BD 1 Delay (ticks)"=w1340, "BD 2 Delay (Ticks)"=w1341, "Next trap write delay (ticks)"=w1342) -> ("error out"=w1259:errorcluster)  [unwired: 1 out]
      n862 = local write "FPGA error out"(w1259) -> ()
    }
    frame #2 {
      # "Initialize some more FPGA settings"
      n863 = local read "Trap Pos FB Monitor\nT1 or T2"() -> (w1364:bool)
      n864 = local read "Trap Pos FB Negate Action"() -> (w1365:bool)
      n865 = local read "Trap Pos. FB Offset Factor"() -> (w1366:i64)
      n866 = local read "Trap Pos. FB Mult Factor"() -> (w1367:i64)
      n867 = local read "Trap Pos. AI1 X Pre-scale"() -> (w1369:u16)
      n868 = local read "Trap Pos FB Int Count"() -> (w1371:u16)
      n869 = local read "Green Laser ON"() -> (w1343:bool)
      n870 = local read "Neg. TTrig FPGA"() -> (w1372:bool)
      n871 = local read "Trap Pos. FB Range"() -> (w1348:T18)
      n872 = local read "Trap Pos. FB Gains"() -> (w1349:T17)
      n873 = local read "Dynamic Force FB (ronen)"() -> (w1350:bool)
      n874 = Multiply(x="Green Intensity % (FB OFF)", y=655.35) -> (x*y=w1358:dbl)
      n875 = Multiply(x="Red FB Setpoint (mV)", y=3.2767) -> (x*y=w1380:dbl)
      n876 = Multiply(x="Red Intensity % (FB OFF)", y=655.35) -> (x*y=w1384:dbl)
      n877 = Unbundle By Name("Red FB Gains") -> ("proportional gain (Kc)"=w1389:i16, "integral gain (Kc*Ts/Ti)"=w1390:i16, "derivative gain (Kc*Td/Ts)"=w1391:i16)
      n878 = Multiply(x="Green FB Setpoint (mV)", y=3.2767) -> (x*y=w1361:dbl)
      n879 = To Unsigned Word Integer(number=w1358) -> (unsigned 16bit integer=w1360:u16)
      n880 = To Unsigned Word Integer(number=w1384) -> (unsigned 16bit integer=w1387:u16)
      n881 = To Word Integer(number=w1380) -> (16bit integer=w1383:i16)
      n882 = local read "Differential FB?"() -> (w1374:bool)
      n883 = To Word Integer(number=w1361) -> (16bit integer=w1363:i16)
      n884 = local read "Laser interlacing mode"() -> (w1346:enum32{"Laser ON", "Laser OFF", "Interlace"})
      n885 = local read "Invert laser interlacing"() -> (w1347:bool)
      n886 = Unbundle By Name("Green FB Gains") -> ("proportional gain (Kc)"=w1377:i16, "integral gain (Kc*Ts/Ti)"=w1378:i16, "derivative gain (Kc*Td/Ts)"=w1379:i16)
      n887 = Select(t=w1346, s=w1343, f=enum32{"Laser ON", "Laser OFF", "Interlace"}."Laser OFF" ("Green laser mode")) -> (s? t:f=w1345:enum32{"Laser ON", "Laser OFF", "Interlace"})
      n888 = local read "FPGA error out"() -> (w1351:errorcluster)
      n889 = xnode "Read/Write Control"("FPGA VI Reference In"=w1353, "error in"=w1351, "Invert GI"=w1347, "Invert GI 2"=w1347, "Invert RI"=w1347, "Invert RI 2"=w1347, "Operating Mode"=w1345, "Operating Mode 2"=w1345, "Red Laser Operating Mode"=w1345, "RI Operating Mode 2"=w1345, "P3"=w1377, "I3"=w1378, "D3"=w1379, "Green FB Setpoint"=w1363, "Green FB On/Off"="Green FB On/Off", "Current Out"=w1360, "Green int current ON count adj"="Green int current ON count adj", "Trap Pos FB Monitor T1 or T2"=w1364, "Trap Pos FB Negate Action"=w1365, "Trap Pos. FB Offset Factor"=w1366, "Trap Pos. FB Mult Factor"=w1367, "Force feedback"=FALSE, "AI1 X Scale"=w1369, "Trap Pos to FIFO"=TRUE, "Trap Pos FB Int Count"=w1371, "TTrig Negate Pos"=w1372, "FB Trig Integrate"="FB Trig Integrate", "Diff FB Measurement?"=w1374, "Negate Diff?"="Negate Diff?", "Trap pos. FB Range"=w1348, "Trap Pos. FB Gains"=w1349, "Red FB Setpoint"=w1383, "RI Current Out"=w1387, "P4"=w1389, "I4"=w1390, "D4"=w1391, "Red FB On/Off"="Red FB On/Off", "Dynamic Force FB (Ronen)"=w1350) -> ("error out"=w1352:errorcluster)  [unwired: 1 out]
      n890 = local write "FPGA error out"(w1352) -> ()
    }
    frame #3 {
      # "Initialize more settings. Should stop using event loops to initialize."
      # "What are these?"
      n891 = local write "Offset (nm)"(0.0 ("Offset (nm)")) -> ()
      n892 = local write "Bead Mean (nm)"(0.0 ("Bead Mean (nm)")) -> ()
      n893 = stacked-sequence {
        frame #0 {
          w1395 = T42."empty" ("mode")
          # "Clear external fluorescence triggering FIFO"
          # "APD loop counts"
          # "Fluorescence loop counts (rates)"
          n894 = local read "APD Integration Time (s)"() -> (w1397:dbl)
          n895 = local read "Interlace ON count"() -> (w1398:u16)
          n896 = call "Smart Buffer (DBL) 1.vi"("mode"=w1395) -> ()  [unwired: 5 in, 6 out]
          n897 = call "Smart Buffer (DBL) 2.vi"("mode"=w1395) -> ()  [unwired: 5 in, 6 out]
          n898 = property on="APD Integration Time (s)" class="DigNum (strict)"("Val(Sgnl)"=w1397) -> ()  [unwired: 2 in, 2 out]
          n899 = property on="Interlace ON count" class="DigNum (strict)"("Val(Sgnl)"=w1398) -> ()  [unwired: 2 in, 2 out]
          "Number of APDs" <- 3.0 ("Number of APDs")
        }
        frame #1 {
          # "Number of APDs affects\nAPD DMA transfer"
          # "General settings for all lasers:"
          # "And includes all laser\nON/OFF settings"
          # "Fluorescent lasers settings:"
          # "Blue laser settings:"
          n900 = local read "Laser interlacing mode"() -> (w1400:enum32{"Laser ON", "Laser OFF", "Interlace"})
          n901 = local read "Invert laser interlacing"() -> (w1399:bool)
          n902 = local read "Blue FB On/Off"() -> (w1401:bool)
          n903 = property on="Blue FB On/Off" class="Bool (strict)"("Val(Sgnl)"=w1401) -> ()  [unwired: 2 in, 2 out]
